vi "坐标旋转(标量）.vi"(8 "Error In":errorcluster caption="错误输入", 10 "dθ（度）":dbl, 11 "输入点":T1 caption="点（双精度）") -> (0 "Error Out":errorcluster caption="错误输出", 3 "输出点":T1 caption="点（双精度）")   [LabVIEW 2012, in "几何工具.lvlib"]
uses:
  <vilib>/Utility/miscctls.llb/LVPointDoubleTypeDef.ctl
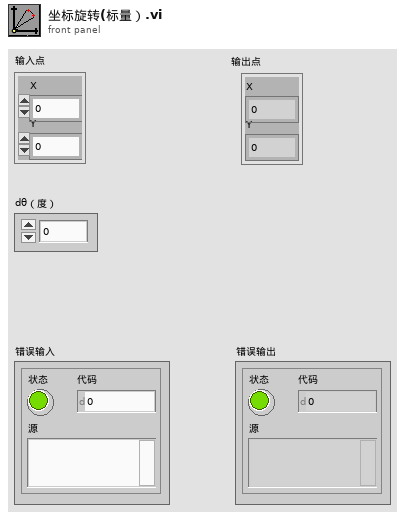
[diagram p1: front panel]
types:
  T1 = typedef "LVPointDoubleTypeDef.ctl" = cluster{"X":dbl, "Y":dbl}
  T2 = typedef "几何工具.lvlib/极坐标.ctl" = cluster{"R":dbl, "θ":dbl}
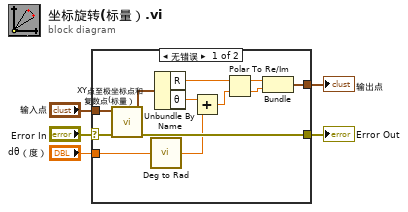
[diagram p0: block diagram]
diagram:
  n1 = case shown="无错误" "Error In" {
    selector: "Error In" -> [w16 w19]
    tunnel: [w8 w19] -> w4
    tunnel: "输入点" -> [w17 w18]
    tunnel: "dθ（度）" -> [w14 _]
    tunnel: [w9 w18] -> w1
    frame No Error {
      n2 = call "XY点至极坐标点和复数点(标量）.vi"("Error In"=w16, "点"=w17) -> ("Error Out"=w8:errorcluster, "极坐标点"=w15:T2)  [unwired: 7 in, 1 out]
      n3 = call-poly "Deg to Rad.vi"("degree"=w14) -> ("radian"=w6:dbl)
      n4 = Unbundle By Name(w15) -> ("R"=w13:dbl, "θ"=w12:dbl)
      n5 = Add(x=w12, y=w6) -> (x+y=w7:dbl)
      n6 = Polar To Re/Im(2:w7, 3:w13) -> (0:w10:dbl, 1:w11:dbl)
      n7 = Bundle(w11, w10) -> (w9:cluster{dbl, dbl})  [unwired: 1 in]
    }
    frame Error {
    }
  }
  "Error Out" <- w4
  "输出点" <- w1
